vi "Read Element of Array of Motor Configuration Objs.vi"(8 "error in (no error)":errorcluster, 10 "index":i32, 11 "MotionSystem Configuration in":refnum<class "MotionSystem Configuration.lvclass">) -> (0 "error out":errorcluster, 2 "Hardware.lvlib:Motor.lvlib:Motor Configuration.lvclass":refnum<class "Motor Configuration.lvclass">, 3 "MotionSystem Configuration out":refnum<class "MotionSystem Configuration.lvclass">)   [LabVIEW 2016, in "MotionSystem.lvlib" / "MotionSystem Configuration.lvclass"]
uses:
  <userlib>/Common Components/Hardware/Abstract System/MotionSystem/MotionSystem Config/MotionSystem Configuration.lvclass
  <userlib>/Common Components/Hardware/Motor/Motor Config/Motor Configuration.lvclass
  <userlib>/Common Components/Hardware/Abstract System/MotionSystem/MotionSystem Config/MotionSystem Configuration.lvclass/MotionSystem Configuration.ctl
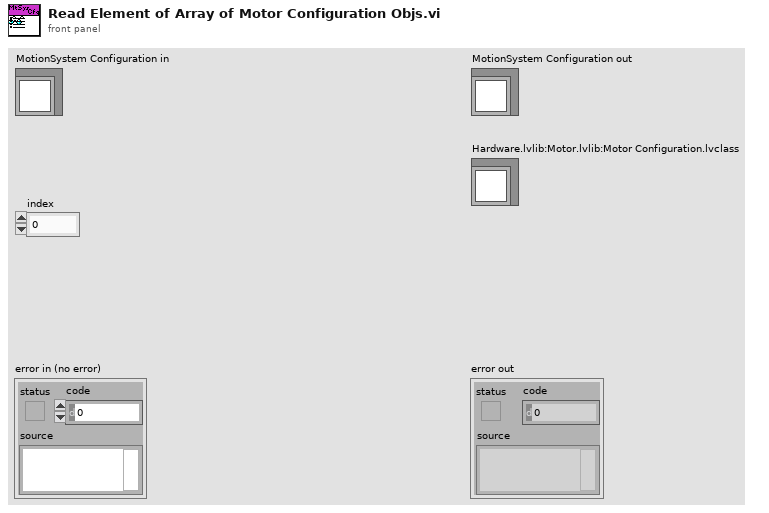
[diagram p1: front panel]
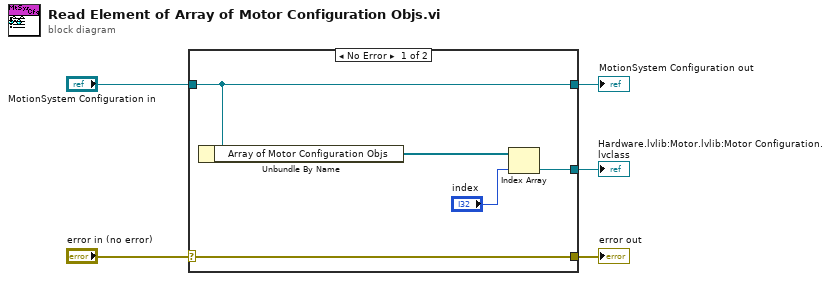
[diagram p0: block diagram]
diagram:
  n1 = case shown="No Error" "error in (no error)" {
    selector: "error in (no error)" -> [w10 w11]
    tunnel: [w10 w11] -> w4
    tunnel: [w9 w12] -> w2
    tunnel: "MotionSystem Configuration in" -> [w9 w12]
    tunnel: [w6 _] -> w1
    frame No Error {
      n2 = Unbundle By Name(w9) -> ("Array of Motor Configuration Objs"=w8:refnum<class "Motor Configuration.lvclass">[])
      n3 = Index Array(array=w8, index="index") -> (element=w6:refnum<class "Motor Configuration.lvclass">)
    }
    frame Error {
    }
  }
  "error out" <- w4
  "MotionSystem Configuration out" <- w2
  "Hardware.lvlib:Motor.lvlib:Motor Configuration.lvclass" <- w1
